vi "RSZVB Set Logical Port Differential Ref Impedance.vi"(6 "Real (100 Ohm)":dbl=100.0 format="%^.3e", 7 "Imaginary (0 Ohm)":dbl format="%^.3e", 8 "error in (no error)":errorcluster {"code" format="%.0x"}, 9 "Port (1)":i32=1, 10 "Channel (1)":i32=1, 11 "VISA session":refnum<visa-resource-name>) -> (0 "error out":errorcluster {"code" format="%.0x"}, 3 "dup VISA session":refnum<visa-resource-name>)   [LabVIEW 2011]
doc: "This VI specifies the complex differential mode reference impedance for the balanced (logical) port numbered <log_port>. \n\nRemote-control command(s):\n[SENSe<Ch>:]LPORt<log_port>:ZDIFferent <real>[, <imaginary>]"
uses:
  _utility/RSZVB Global Data.vi
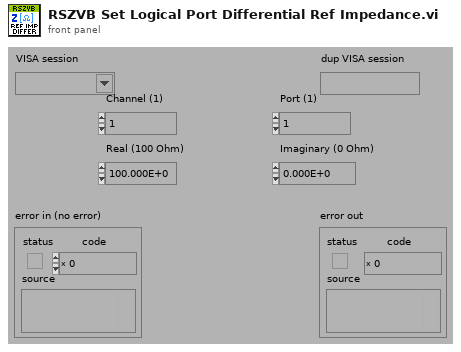
[diagram p1: front panel]
types:
  T1 = cluster{"Error Checking (T: On)":bool, "Installed Options":string[], "Data Valid?":bool, "Ports":i32, "Model":string[], "Option Checking (T: On)":bool}[]
  T2 = cluster{"Error Checking (T: On)":bool, "Installed Options":string[], "Data Valid?":bool, "Ports":i32, "Model":string[], "Option Checking (T: On)":bool}
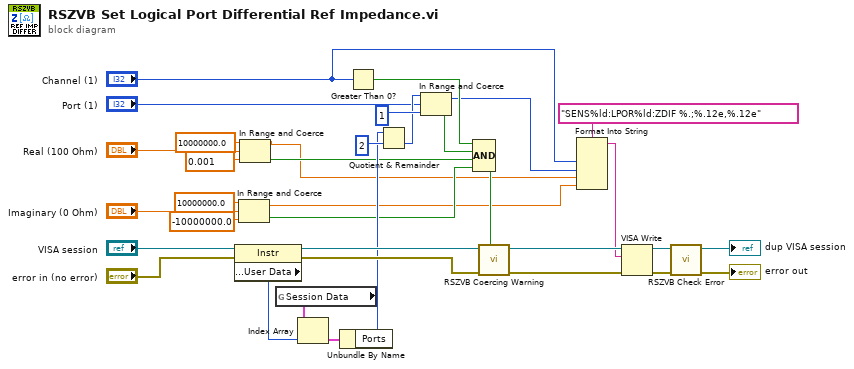
[diagram p0: block diagram]
diagram:
  n1 = property class="Instr"(reference="VISA session", error in="error in (no error)") -> (reference out=w34:refnum<visa-resource-name>, error out=w33:errorcluster, "General Settings:User Data"=w32:u32)
  n2 = In Range and Coerce(upper limit=10000000.0 ("lower limit"), x="Imaginary (0 Ohm)", lower limit=-10000000.0) -> (coerced(x)=w9:dbl, In Range?=w18:bool)
  n3 = In Range and Coerce(upper limit=10000000.0 ("lower limit"), x="Real (100 Ohm)", lower limit=0.001) -> (coerced(x)=w10:dbl, In Range?=w19:bool)
  n4 = global read "RSZVB Global Data.vi" "Session Data"() -> (w31:T1)
  n5 = Index Array(array=w31, index=w32) -> (element=w30:T2)
  n6 = Unbundle By Name(w30) -> ("Ports"=w24:i32)
  n7 = Greater Than 0?(x="Channel (1)") -> (x > 0?=w29:bool)
  n8 = Quotient & Remainder(x=w24, y=2) -> (floor(x/y)=w21:i32)  [unwired: 1 out]
  n9 = In Range and Coerce(upper limit=w21, x="Port (1)", lower limit=1) -> (coerced(x)=w11:i32, In Range?=w20:bool)
  n10 = Compound Arithmetic op=AND(w29, w20, w19, w18) -> (w28:bool)
  n11 = call "RSZVB Coercing Warning.vi"("In Range?"=w28, "error in (no error)"=w33, "VISA session"=w34) -> ("error out"=w15:errorcluster, "dup VISA session"=w14:refnum<visa-resource-name>)  [unwired: 7 in]
  n12 = Format Into String(format string="SENS%ld:LPOR%ld:ZDIF %.;%.12e,%.12e", "Channel (1)", w11, w10, w9) -> (resulting string=w13:string)  [unwired: 2 in, 1 out]
  n13 = VISA Write(VISA resource name=w14, write buffer=w13, error in (no error)=w15) -> (VISA resource name out=w17:refnum<visa-resource-name>, error out=w16:errorcluster)  [unwired: 1 out]
  n14 = call "RSZVB Check Error.vi"("error in (no error)"=w16, "VISA session"=w17) -> ("error out"=→"error out":errorcluster, "dup VISA session"=→"dup VISA session":refnum<visa-resource-name>)  [unwired: 8 in]
